vi "ParseVeriStandProtocolLog.vi"(8 "error in (no error)":errorcluster, 10 "Path":path=path "C:/LVLibrary/XNET/XCP_otherID/XCP_OtherDTOID/ECUMCLog/XCP or CCP Master_Protocol_Log.txt", 11 "DAQList in":refnum<class "DAQList.lvclass">) -> (0 "error out":errorcluster, 2 "CAN Frames":T1[](array[typedef]) {"payload" format="%x"; "timestamp" format="%<%.7X\n%x>T"; "type" items=["CAN Data"=0, "CAN Remote"=1, "CAN Bus Error"=2, "CAN 2.0 Data"=8, "CAN FD Data"=16, "CAN FD+BRS Data"=24, "J1939 Data"=192, "Delay"=224, "Log Trigger"=225, "Start Trigger"=226]; "identifier" format="%x"}, 3 "DAQList out":refnum<class "DAQList.lvclass">)   [LabVIEW 2019, in "XCP_DaqDtoId.lvlib" / "DAQList.lvclass"]
uses:
  DAQList.lvclass
  <vilib>/xnet/xnet.llb/XNET Frame CAN.ctl
  <vilib>/xnet/xnet.llb/XNET Frame Type CAN.ctl
  <vilib>/Utility/file.llb/Read Delimited Spreadsheet (string).vi
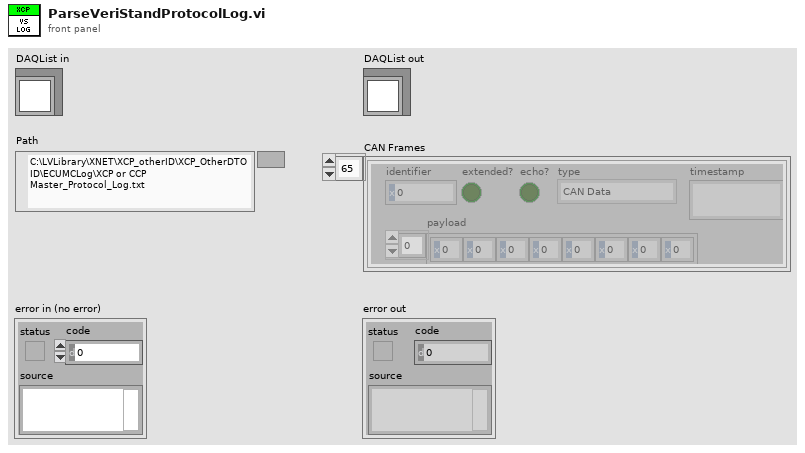
[diagram p1: front panel]
types:
  T1 = typedef "XNET Frame CAN.ctl" = cluster{"timestamp":timestamp, "payload":u8[], "identifier":u32, "type":T2, "extended?":bool, "echo?":bool}
  T2 = typedef "XNET Frame Type CAN.ctl" = u8
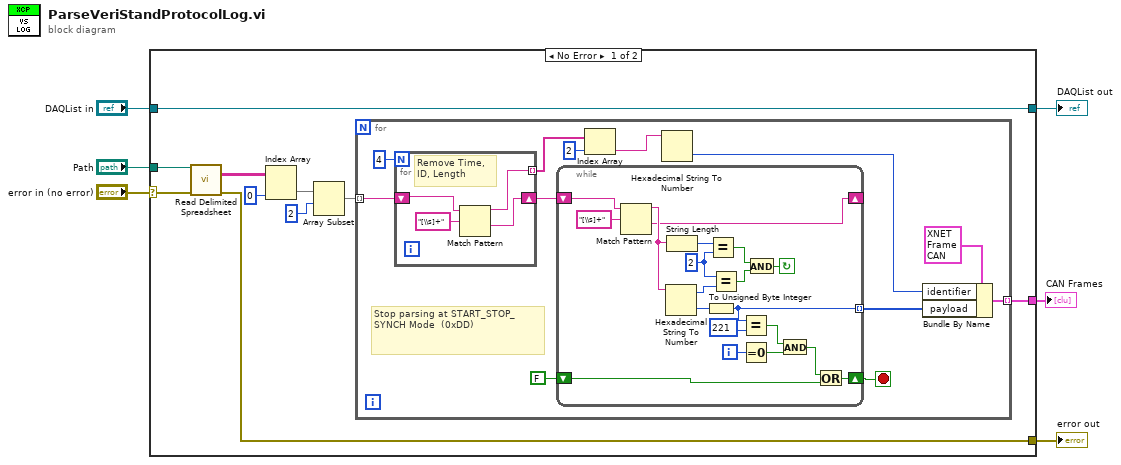
[diagram p0: block diagram]
diagram:
  n1 = case shown="No Error" "error in (no error)" {
    selector: "error in (no error)" -> [w14 w53]
    tunnel: [w13 w53] -> w5
    tunnel: [w16 w52] -> w3
    tunnel: "DAQList in" -> [w16 w52]
    tunnel: "Path" -> [w15 _]
    tunnel: [w7 _] -> w1
    frame No Error {
      n2 = call-poly <vilib>:"Read Delimited Spreadsheet.vi"("file path (dialog if empty)"=w15, "error in (no error)"=w14) -> ("all rows"=w11:string[][], "error out"=w13:errorcluster)  [unwired: 8 in, 4 out]
      n3 = Index Array(array=w11, index (col)=0 ("disabled index (col)")) -> (element=w9:string[])  [unwired: 1 in]
      n4 = Array Subset(array=w9, index=2) -> (w8:string[])  [unwired: 1 in]
      n5 = for {
        tunnel: w8 -> [w24] mode=indexing
        tunnel: [w23] -> w7 mode=indexing
        stop <- w17 stop-if-true
        # "Stop parsing at START_STOP_SYNCH Mode  (0xDD)"
        n6 = for {
          N: 4 -> [_]
          shift-right: [w49] -> w27
          shift-left: w24 -> [w51]
          tunnel: [w48] -> w22 mode=indexing
          # "Remove Time, ID, Length"
          n7 = Match Pattern(string=w51, regular expression="[\\s]+") -> (before substring=w48:string, after substring=w49:string)  [unwired: 1 in, 2 out]
        }
        n8 = while {
          shift-right: [w38] -> _
          shift-left: w27 -> [w47]
          tunnel: [w35] -> w25 mode=indexing
          shift-right: [w30] -> w17
          shift-left: FALSE -> [w29]
          i -> [w36]
          stop <- w39 continue-if-true
          w43 = 2 ("y")
          n9 = Match Pattern(string=w47, regular expression="[\\s]+") -> (before substring=w44:string, after substring=w38:string)  [unwired: 1 in, 2 out]
          n10 = Hexadecimal String To Number(string=w44) -> (offset past number=w42:i32, number=w37:u32)  [unwired: 2 in]
          n11 = String Length(string=w44) -> (length=w45:i32)
          n12 = To Unsigned Byte Integer(number=w37) -> (unsigned 8bit integer=w35:u8)
          n13 = Equal?(x=w45, y=w43) -> (x = y?=w41:bool)
          n14 = Equal?(x=w43, y=w42) -> (x = y?=w40:bool)
          n15 = Equal?(x=w35, y=u8 221 ("unsigned 8bit integer")) -> (x = y?=w33:bool)
          n16 = Equal To 0?(x=w36) -> (x = 0?=w32:bool)
          n17 = And(x=w41, y=w40) -> (x .and. y?=w39:bool)
          n18 = And(x=w33, y=w32) -> (x .and. y?=w31:bool)
          n19 = Or(x=w31, y=w29) -> (x .or. y?=w30:bool)
        }
        n20 = Index Array(array=w22, index=2) -> (element=w20:string)
        n21 = Hexadecimal String To Number(string=w20) -> (number=w19:u32)  [unwired: 2 in, 1 out]
        n22 = Bundle By Name(cluster=T1 {"timestamp"=timestamp(0 s since 1904-01-01), "payload"=[], "identifier"=0, "type"=0, "extended?"=FALSE, "echo?"=FALSE} ("CAN frame"), "identifier"=w19, "payload"=w25) -> (w23:T1)
      }
    }
    frame Error {
    }
  }
  "error out" <- w5
  "DAQList out" <- w3
  "CAN Frames" <- w1
